vi "CC Data Logging Loop.vi"(11 "user event":refnum<user-event>) -> ()   [LabVIEW 2021]
uses:
  hk-channel-class/HK Table/HK Table.lvclass
  Subsystems/SS cluster Data Queue type.ctl
  CC enum Current Values Action.ctl
  Subsystems/SS cluster New Image Data.ctl
  typedefs/CC cluster Alarm Data.ctl
  typedefs/CC enum Alarm Action.ctl
  typedefs/CC cluster System Settings.ctl
  hk-channel-class/HK Item/HK Item.lvclass
panel:
  out "error out":errorcluster
  in  "error in (no error)":errorcluster
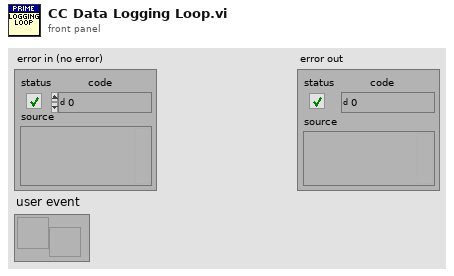
[diagram p1: front panel]
types:
  T1 = cluster{"HK Channels":refnum<class "HK Table.lvclass">, "Data Q":refnum<queue>, "user event":refnum<user-event>}
  T2 = typedef "CC enum Current Values Action.ctl" = enum16{"Init", "Write Item", "Write Array", "Read Item", "Read Array", "Read All", "Add Channels", "New File", "Add Message", "Get Current Values", "Close"}
  T3 = typedef "SS cluster New Image Data.ctl" = cluster{"Frame number":i32, "Detector #":u16, "FITS file":path, "File size":i64}
  T4 = typedef "SS cluster Data Queue type.ctl" = cluster{"Source":string, "Type":string, "Data":variant}
  T5 = typedef "CC enum Alarm Action.ctl" = enum16{"Init", "Add Alarm", "Get Alarms", "Clear Alarm", "Clear All Alarms"}
  T6 = typedef "CC cluster Alarm Data.ctl" = cluster{"Measured Value":dbl, "Alarm Low":dbl, "Alarm High":dbl, "Message":string, "Source":string}
  T7 = typedef "CC cluster System Settings.ctl" = cluster{"HK Table Name":string, "Images Folder":path, "Obs File":path}
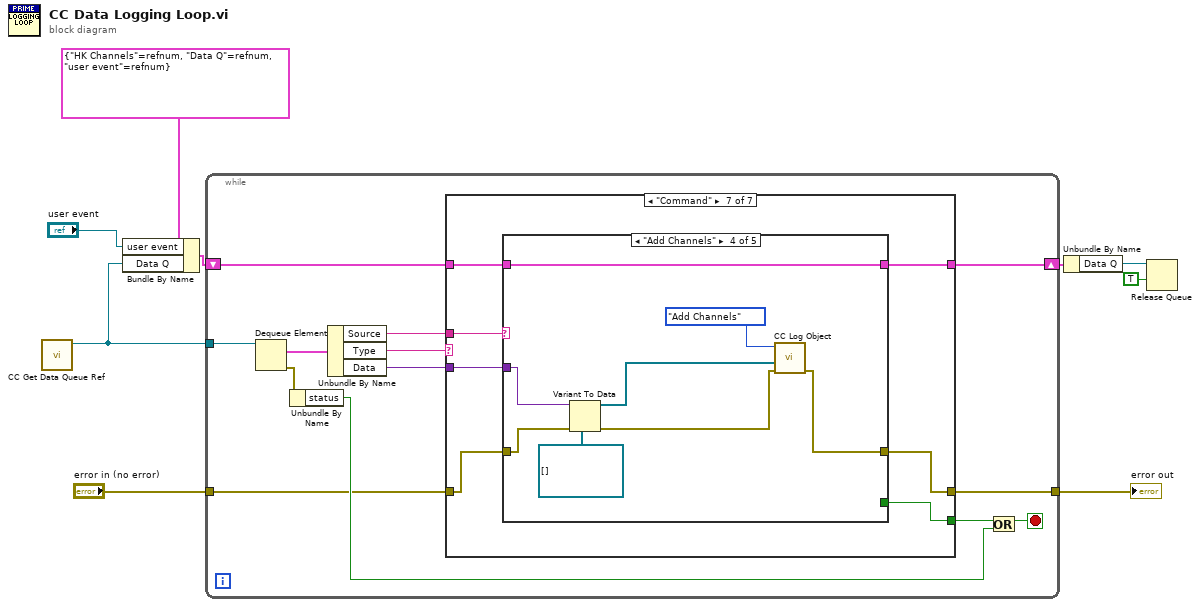
[diagram p0: block diagram]
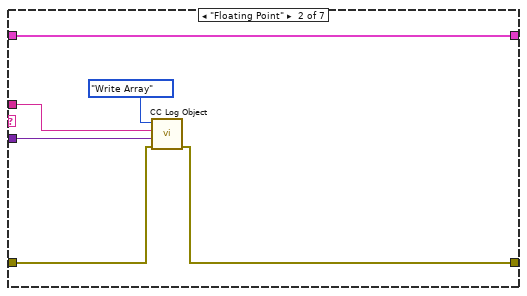
[diagram p3: hidden frame]
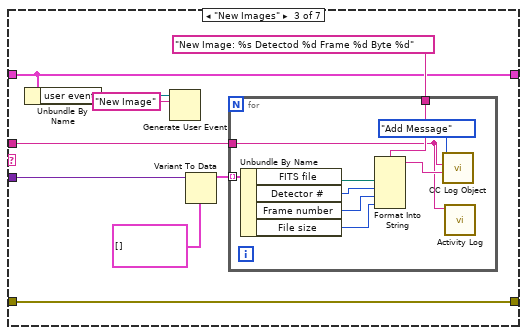
[diagram p4: hidden frame]
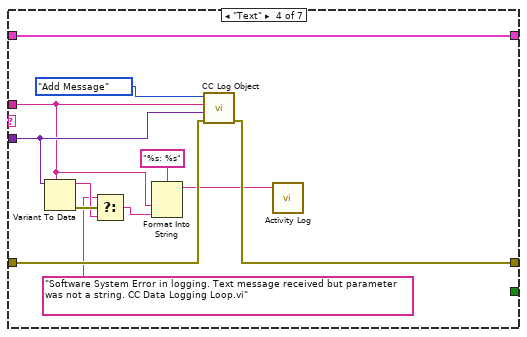
[diagram p5: hidden frame]
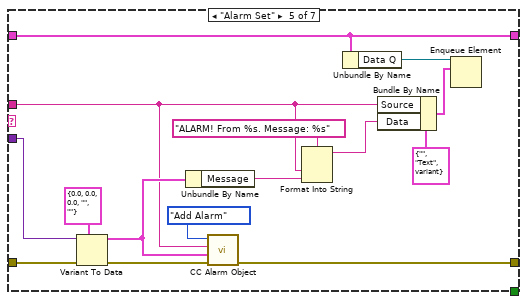
[diagram p6: hidden frame]
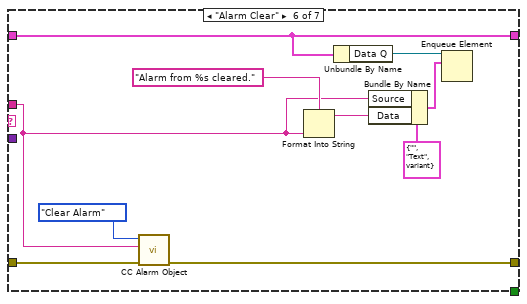
[diagram p7: hidden frame]
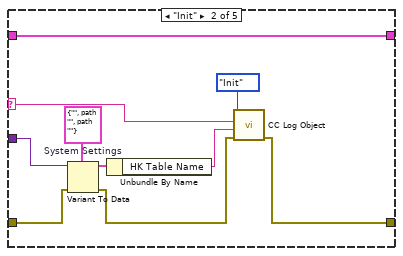
[diagram p9: hidden frame]
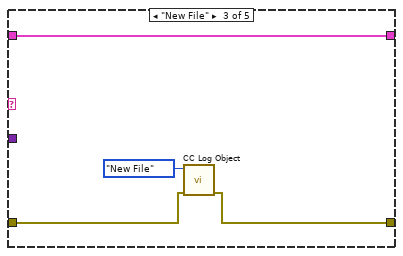
[diagram p10: hidden frame]
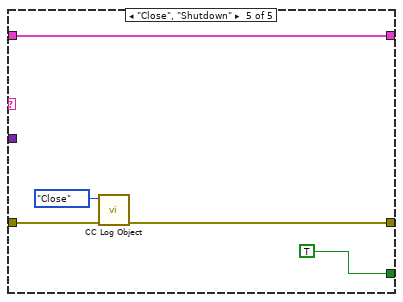
[diagram p11: hidden frame]
diagram:
  n1 = call "CC Get Data Queue Ref.vi"() -> ("Data Q"=w7:refnum<queue>)  [unwired: 10 in, 1 out]
  n2 = Bundle By Name(cluster=T1 {"HK Channels"=refnum, "Data Q"=refnum, "user event"=refnum}, "user event"="user event", "Data Q"=w7) -> (w5:T1)
  n3 = while {
    tunnel: w7 -> [w22]
    shift-right: [w12] -> w4
    shift-left: w5 -> [w16]
    tunnel: "error in (no error)" -> [w17]
    tunnel: [w11] -> w8
    stop <- w20 stop-if-true
    n4 = Dequeue Element(queue=w22) -> (element=w21:T4, error out=w19:errorcluster)  [unwired: 2 in, 2 out]
    n5 = Unbundle By Name(w19) -> ("status"=w18:bool)
    n6 = Unbundle By Name(w21) -> ("Source"=w14:string, "Type"=w15:string, "Data"=w13:variant)
    n7 = case shown="\"Command\"" w15 {
      tunnel: w13 -> [_ w28 w39 w56 w75 _ w89]
      tunnel: w16 -> [w24 w27 w33 w59 w69 w77 w92]
      tunnel: [w24 w27 w33 w59 w69 w77 w91] -> w12
      tunnel: w14 -> [_ w29 w35 w54 w63 w76 w86]
      tunnel: w17 -> [w23 w26 w34 w58 w72 w83 w90]
      tunnel: [w23 w25 w34 w57 w70 w84 w88] -> w11
      tunnel: [_ _ _ _ _ _ w87] -> w10
      frame "False", Default {
      }
      frame "Floating Point" {
        n8 = call "CC Log Object.vi"("error in (no error)"=w26, "Data"=w28, "Source"=w29, "Action"=CC_enum_Current_Values_Action."Write Array") -> ("error out"=w25:errorcluster)  [unwired: 5 in, 2 out]
      }
      frame "New Images" {
        n9 = Unbundle By Name(w33) -> ("user event"=w32:refnum<user-event>)
        n10 = Generate User Event(user event=w32, event data cluster="New Image" ("event data")) -> ()  [unwired: 2 in, 2 out]
        n11 = Variant To Data(type=T3[] [], Variant=w39) -> (data=w37:T3[])  [unwired: 1 in, 1 out]
        n12 = for {
          tunnel: w37 -> [w48] mode=indexing
          tunnel: "New Image: %s Detectod %d Frame %d Byte %d" ("format string") -> [w47]
          tunnel: w35 -> [w40]
          n13 = Unbundle By Name(w48) -> ("FITS file"=w46:path, "Detector #"=w45:u16, "Frame number"=w44:i32, "File size"=w43:i64)
          n14 = Format Into String(format string=w47, w46, w45, w44, w43) -> (resulting string=w41:string)  [unwired: 2 in, 1 out]
          n15 = call "CC Log Object.vi"("Data"=w41, "Source"=w40, "Action"=CC_enum_Current_Values_Action."Add Message") -> ()  [unwired: 6 in, 3 out]
          n16 = call "Activity Log.vi"("Message Log Entry"=w40) -> ()  [unwired: 9 in, 2 out]
        }
      }
      frame "Text" {
        n17 = Variant To Data(type=w54, Variant=w56) -> (data=w51:string, error out=w52:errorcluster)  [unwired: 1 in]
        n18 = Select(t="Software System Error in logging. Text message received but parameter was not a string. CC Data Logging Loop.vi", s=w52, f=w51) -> (s? t:f=w50:string)
        n19 = Format Into String(format string="%s: %s", w54, w50) -> (resulting string=w53:string)  [unwired: 2 in, 1 out]
        n20 = call "CC Log Object.vi"("error in (no error)"=w58, "Data"=w56, "Source"=w54, "Action"=CC_enum_Current_Values_Action."Add Message") -> ("error out"=w57:errorcluster)  [unwired: 5 in, 2 out]
        n21 = call "Activity Log.vi"("Message Log Entry"=w53) -> ()  [unwired: 9 in, 2 out]
      }
      frame "Alarm Set" {
        n22 = Variant To Data(error in=w72, type=T6 {"Measured Value"=0.0, "Alarm Low"=0.0, "Alarm High"=0.0, "Message"="", "Source"=""}, Variant=w75) -> (data=w66:T6, error out=w71:errorcluster)
        n23 = Unbundle By Name(w66) -> ("Message"=w62:string)
        n24 = call "CC Alarm Object.vi"("error in (no error)"=w71, "Alarm"=w66, "Source"=w63, "Alarm Action"=CC_enum_Alarm_Action."Add Alarm") -> ("error out"=w70:errorcluster)  [unwired: 5 in, 2 out]
        n25 = Format Into String(format string="ALARM! From %s. Message: %s", w63, w62) -> (resulting string=w61:string)  [unwired: 2 in, 1 out]
        n26 = Unbundle By Name(w69) -> ("Data Q"=w68:refnum<queue>)
        n27 = Bundle By Name(cluster=T4 {"Source"="", "Type"="Text", "Data"=variant} ("element"), "Source"=w63, "Data"=w61) -> (w65:T4)
        n28 = Enqueue Element(queue=w68, element=w65) -> ()  [unwired: 2 in, 3 out]
      }
      frame "Alarm Clear" {
        n29 = call "CC Alarm Object.vi"("error in (no error)"=w83, "Source"=w76, "Alarm Action"=CC_enum_Alarm_Action."Clear Alarm") -> ("error out"=w84:errorcluster)  [unwired: 6 in, 2 out]
        n30 = Format Into String(format string="Alarm from %s cleared.", w76) -> (resulting string=w78:string)  [unwired: 2 in, 1 out]
        n31 = Unbundle By Name(w77) -> ("Data Q"=w82:refnum<queue>)
        n32 = Bundle By Name(cluster=T4 {"Source"="", "Type"="Text", "Data"=variant} ("element"), "Source"=w76, "Data"=w78) -> (w80:T4)
        n33 = Enqueue Element(queue=w82, element=w80) -> ()  [unwired: 2 in, 3 out]
      }
      frame "Command" {
        n34 = case shown="\"Add Channels\"" w86 {
          selector: w86 -> [_ w101 _ _ _]
          tunnel: w92 -> [w93 w99 w108 w113 w121]
          tunnel: [w93 w99 w108 w113 w121] -> w91
          tunnel: w90 -> [w94 w95 w105 w111 w119]
          tunnel: [w94 w98 w106 w110 w118] -> w88
          tunnel: [_ _ _ _ TRUE] -> w87
          tunnel: w89 -> [_ w97 _ w109 _]
          frame "False", Default {
          }
          frame "Init" {
            w104 = T7 {"HK Table Name"="", "Images Folder"=path "", "Obs File"=path ""}  # System Settings
            n35 = Variant To Data(error in=w95, type=w104, Variant=w97) -> (data=w103:T7, error out=w96:errorcluster)
            n36 = Unbundle By Name(w103) -> ("HK Table Name"=w100:string)
            n37 = call "CC Log Object.vi"("error in (no error)"=w96, "Data"=w100, "Source"=w101, "Action"=CC_enum_Current_Values_Action."Init") -> ("error out"=w98:errorcluster)  [unwired: 5 in, 2 out]
          }
          frame "New File" {
            n38 = call "CC Log Object.vi"("error in (no error)"=w105, "Action"=CC_enum_Current_Values_Action."New File") -> ("error out"=w106:errorcluster)  [unwired: 7 in, 2 out]
          }
          frame "Add Channels" {
            n39 = Variant To Data(error in=w111, type=refnum<class "HK Item.lvclass">[] [], Variant=w109) -> (data=w114:refnum<class "HK Item.lvclass">[], error out=w112:errorcluster)
            n40 = call "CC Log Object.vi"("error in (no error)"=w112, "Data"=w114, "Action"=CC_enum_Current_Values_Action."Add Channels") -> ("error out"=w110:errorcluster)  [unwired: 6 in, 2 out]
          }
          frame "Close", "Shutdown" {
            n41 = call "CC Log Object.vi"("error in (no error)"=w119, "Action"=CC_enum_Current_Values_Action."Close") -> ("error out"=w118:errorcluster)  [unwired: 7 in, 2 out]
          }
        }
      }
    }
    n42 = Or(x=w10, y=w18) -> (x .or. y?=w20:bool)
  }
  "error out" <- w8
  n43 = Unbundle By Name(w4) -> ("Data Q"=w3:refnum<queue>)
  n44 = Release Queue(queue=w3, force destroy? (F)=TRUE) -> ()  [unwired: 1 in, 3 out]
